vi "MH_MeasurementDone.vi"(8 "error in (no error)":errorcluster, 9 "Coincidences":u32[](array[numeric]), 10 "MH_Meas_Error":errorcluster, 11 "SinglePhotonInterferenceUI in":refnum<class "SinglePhotonInterferenceUI.lvclass">) -> (0 "error out":errorcluster, 3 "SinglePhotonInterferenceUI out":refnum<class "SinglePhotonInterferenceUI.lvclass">)   [LabVIEW 2023, in "SinglePhoton Library.lvlib" / "SinglePhotonInterferenceUI.lvlib" / "SinglePhotonInterferenceUI.lvclass"]
uses:
  SinglePhotonInterferenceUI.lvclass
  SinglePhotonInterferenceUI.lvclass/SinglePhotonInterferenceUI.ctl
panel:
  in  "event data":T1
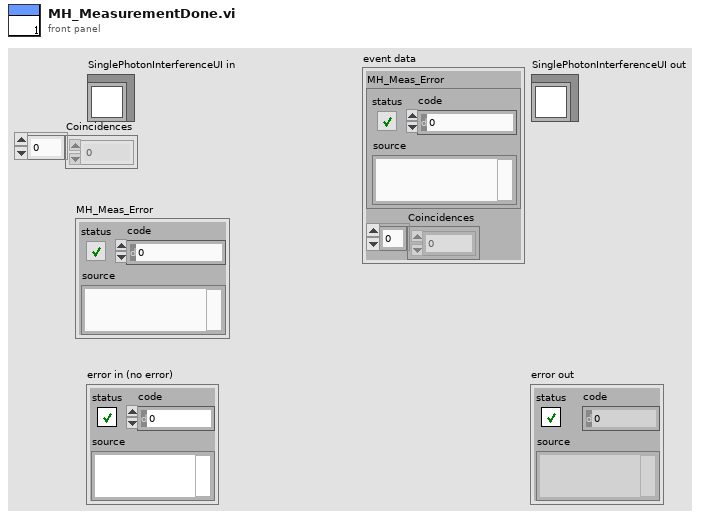
[diagram p1: front panel]
types:
  T1 = cluster{"MH_Meas_Error":errorcluster, "Coincidences":i32[]}
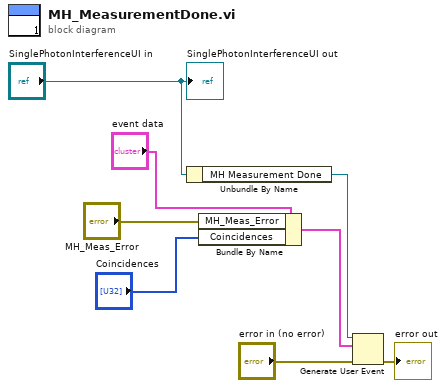
[diagram p0: block diagram]
diagram:
  n1 = Unbundle By Name("SinglePhotonInterferenceUI in") -> ("MH Measurement Done"=w7:refnum<user-event>)
  n2 = Bundle By Name(cluster="event data", "MH_Meas_Error"="MH_Meas_Error", "Coincidences"="Coincidences") -> (w4:T1)
  n3 = Generate User Event(user event=w7, event data cluster=w4, error in="error in (no error)") -> (error out=→"error out":errorcluster)  [unwired: 1 in, 1 out]
  "SinglePhotonInterferenceUI out" <- "SinglePhotonInterferenceUI in"
